vi "Pre Launch Init.vi"(11 "NI_DAQmx(Linear) in":refnum<class "NI_DAQmx(Linear).lvclass">) -> (0 "error out":errorcluster, 3 "NI_DAQmx(Linear) out":refnum<class "NI_DAQmx(Linear).lvclass">)   [LabVIEW 2025, in "NI_DAQmx(Linear).lvclass"]
doc: "<p>(<strong>Filename</strong>: <span class=\"dnl\">Actor Framework.lvlib:Actor.lvclass:Pre Launch Init.vi</span>)</p>\n<p>Defines behavior that occurs after the <a href=\"nihelplauncher://docs/csh?context=lvcore_lvcomm_af_launch_nested_actor\">Launch Nested Actor</a> method is invoked but before the actor's Actor Core method begins running.</p>\n<p>By default, this method does nothing. A descendant class may override it to define behavior.</p>"
uses:
  NI_DAQmx(Linear).lvclass
  NI_DAQmx(Linear).lvclass/NI_DAQmx(Linear).ctl
  Write task.vi
  <vilib>/DAQmx/create/channels.llb/DAQmx Create Channel (CI-Position-Linear Encoder).vi
  <vilib>/DAQmx/configure/timing.llb/DAQmx Timing (Sample Clock).vi
  DAQ_Abstr/Task_Type/Linear_Task/Linear_Task/Linear_Task.lvclass
  <resource>/objmgr/daqmx.rc
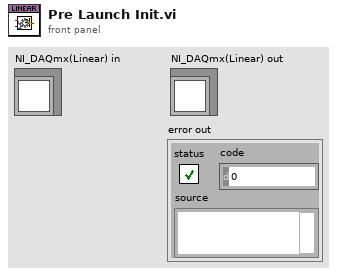
[diagram p1: front panel]
types:
  T1 = typedef "DAQ_Module.lvlib/DAQ_Module.lvclass/DAQ_Task_Config.ctl" = cluster{"Drive":T2, "TaskType":T3, "PhysicalChannels":string, "SampleRateConfiguration":T4, "ChannelConfig":map{string, cluster{"PhysicalChannels":string, "Config":string}}, "Enable":bool, "ShowPanel":bool}
  T2 = typedef "DAQ_Module.lvlib/DAQ_Module.lvclass/DAQ_HW_Type.ctl" = enum16{"NI_DAQmx", "Simulated_DAQ"}
  T3 = typedef "DAQ_Module.lvlib/DAQ_Module.lvclass/DAQ_Task_Type.ctl" = enum16{"AI", "Linear", "Angular", "AO"}
  T4 = typedef "DAQ_Module.lvlib/DAQ_Module.lvclass/DAQ_SampleRateConfig.ctl" = cluster{"SampleRate":dbl, "SamplesPerChannel":u32, "SamplesPerRead":i32, "SampleMode":i32, "Clock Source":string}
  T5 = typedef "DAQ_Module.lvlib/DAQ_Module.lvclass/DAQ_Linear_Task_Config.ctl" = cluster{"decoding type":i32, "units":i32, "distance per pulse":dbl, "initial position":dbl, "z index enable":bool, "z index value":dbl, "z index phase":i32, "CI_Encoder_A_InputTerm":string, "CI_Encoder_B_InputTerm":string, "CI_Encoder_Z_InputTerm":string}
  T6 = map{string, cluster{"Name":string, "Data out":T5}}
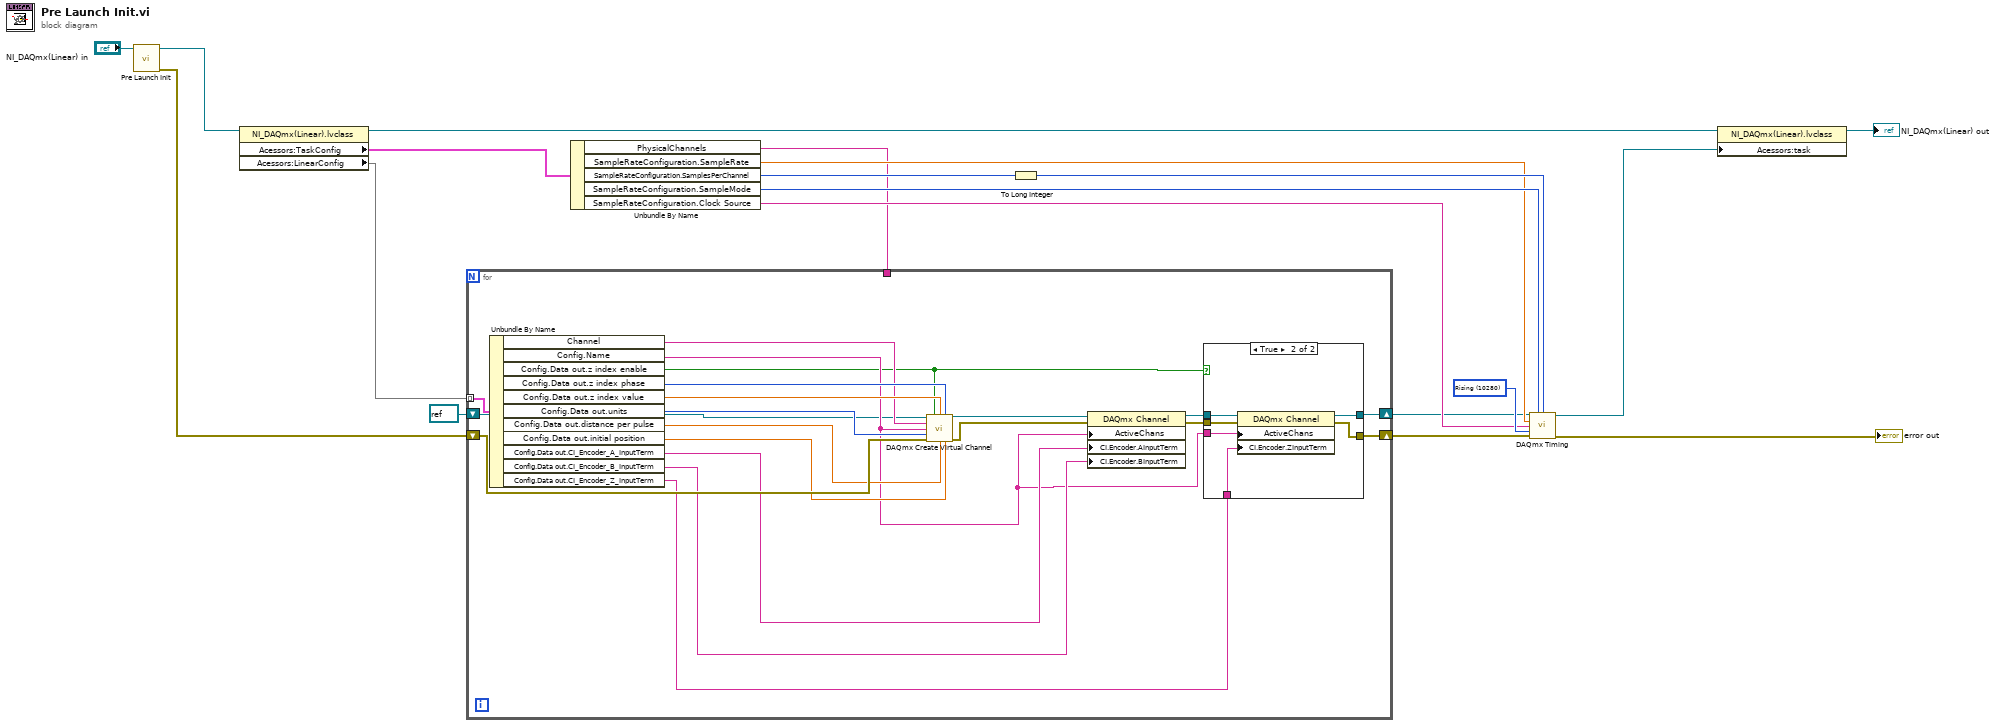
[diagram p0: block diagram]
diagram:
  w11 = 10280 items=["Rising"=10280, "Falling"=10171] ("active edge")
  n1 = call-parent "Pre Launch Init.vi"("Task_Abstr in"="NI_DAQmx(Linear) in") -> ("error out"=w5:errorcluster, "Task_Abstr out"=w7:refnum<class "NI_DAQmx(Linear).lvclass">)  [unwired: 9 in]
  n2 = property class="NI_DAQmx(Linear).lvclass"(reference=w7) -> (reference out=w18:refnum<class "NI_DAQmx(Linear).lvclass">, "Acessors:TaskConfig"=w16:T1, "Acessors:LinearConfig"=w17:T6)  [unwired: 1 in, 1 out]
  n3 = Unbundle By Name(w16) -> ("PhysicalChannels"=w8:string, "SampleRateConfiguration.SampleRate"=w12:dbl, "SampleRateConfiguration.SamplesPerChannel"=w14:u32, "SampleRateConfiguration.SampleMode"=w15:i32, "SampleRateConfiguration.Clock Source"=w10:string)
  n4 = for {
    tunnel: w17 -> [w39] mode=indexing
    tunnel: w8 -> [_]
    shift-right: [w27] -> w2
    shift-left: w5 -> [w38]
    shift-right: [w29] -> w3
    shift-left: refnum<k21> refnum ("task out") -> [w20]
    n5 = Unbundle By Name(w39) -> ("Channel"=w23:string, "Config.Name"=w22:string, "Config.Data out.z index enable"=w21:bool, "Config.Data out.z index phase"=w37:i32, "Config.Data out.z index value"=w36:dbl, "Config.Data out.units"=w35:i32, "Config.Data out.distance per pulse"=w34:dbl, "Config.Data out.initial position"=w33:dbl, "Config.Data out.CI_Encoder_A_InputTerm"=w26:string, "Config.Data out.CI_Encoder_B_InputTerm"=w25:string, "Config.Data out.CI_Encoder_Z_InputTerm"=w24:string)
    n6 = call-poly <vilib>:"DAQmx Create Virtual Channel.vi"("task in"=w20, "z index enable"=w21, "z index value"=w36, "z index phase"=w37, "counter"=w23, "name to assign"=w22, "units"=w35, "error in"=w38, "distance per pulse"=w34, "initial position"=w33) -> ("task out"=w30:refnum<k21>, "error out"=w28:errorcluster)  [unwired: 4 in]
    n7 = property class="DAQmx Channel"(reference=w30, error in=w28, "ActiveChans"=w22, "CI.Encoder.AInputTerm"=w26, "CI.Encoder.BInputTerm"=w25) -> (reference out=w32:refnum<k21>, error out=w31:errorcluster)
    n8 = case shown="True" w21 {
      tunnel: w32 -> [w41 w47]
      tunnel: w31 -> [w40 w46]
      tunnel: [w40 w45] -> w27
      tunnel: [w41 w44] -> w29
      tunnel: w22 -> [_ w43]
      tunnel: w24 -> [_ w42]
      frame False {
      }
      frame True {
        n9 = property class="DAQmx Channel"(reference=w47, error in=w46, "ActiveChans"=w43, "CI.Encoder.ZInputTerm"=w42) -> (reference out=w44:refnum<k21>, error out=w45:errorcluster)
      }
    }
  }
  n10 = To Long Integer(number=w14) -> (32bit integer=w13:i32)
  n11 = call-poly <vilib>:"DAQmx Timing.vi"("task/channels in"=w3, "sample mode"=w15, "samples per channel"=w13, "rate"=w12, "source"=w10, "active edge"=w11, "error in"=w2) -> ("task out"=w9:refnum<k21>, "error out"=→"error out":errorcluster)  [unwired: 7 in]
  n12 = property class="NI_DAQmx(Linear).lvclass"(reference=w18, "Acessors:task"=w9) -> (reference out=→"NI_DAQmx(Linear) out":refnum<class "NI_DAQmx(Linear).lvclass">)  [unwired: 1 in, 1 out]
